vi "Piezo Calibration Param Set.vi"   [LabVIEW 2016, in "Nanonis Prog Interface.lvlib"]
doc: "<B>Sets the piezo range (m) or sensitivity (m/V) values for all 3 axes (X, Y, Z). </B>\n\nThis is a polymorphic funtion where you can select between sensitivity and range of the scan piezo. \n\n- Nanonis Programming Interface -"
uses:
  Nanonis Prog Interface.lvlib
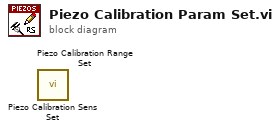
[diagram p0: block diagram]
diagram:
  n1 = call <userlib>:"Piezo Calibration Sens Set.vi"() -> ()  [unwired: 14 in, 2 out]
  n2 = call <userlib>:"Piezo Calibration Range Set.vi"() -> ()  [unwired: 14 in, 2 out]
